vi "Istwerte als Cluster.vi"(8 "error in (no error)":errorcluster caption="Fehler (Eingang, kein Fehler)", 11 "Steuerung PNS Eingang":refnum<class "Steuerung PNS.lvclass">) -> (0 "error out":errorcluster caption="Fehler (Ausgang)", 2 "Cluster":cluster{"UsrVal":u16[], "Alarm":T1, "Regler":T2}, 3 "Steuerung PNS Ausgang":refnum<class "Steuerung PNS.lvclass">)   [LabVIEW 2020, in "Steuerung PNS.lvclass"]
doc: "Gibt die Istwerte von UsrVal, Regler und Alarme als Cluster zurück.\n(zum schreiben in die FGV PNS Istwerte)\nRIW"
uses:
  Steuerung PNS.lvclass
  Alarme.ctl
  Regler.ctl
  Steuerung PNS.lvclass/Steuerung PNS.ctl
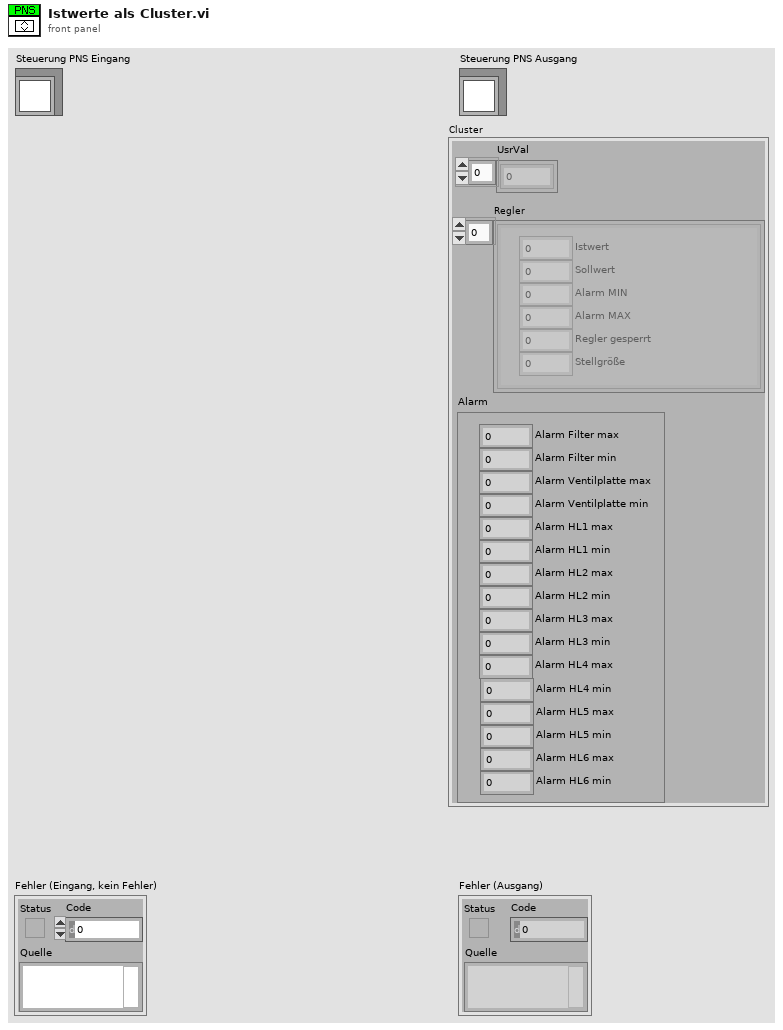
[diagram p1: front panel]
types:
  T1 = typedef "Steuerung PNS.lvclass/Alarme.ctl" = cluster{"Alarm Filter max":u16, "Alarm Filter min":u16, "Alarm Ventilplatte max":u16, "Alarm Ventilplatte min":u16, "Alarm HL1 max":u16, "Alarm HL1 min":u16, "Alarm HL2 max":u16, "Alarm HL2 min":u16, "Alarm HL3 max":u16, "Alarm HL3 min":u16, "Alarm HL4 max":u16, "Alarm HL4 min":u16, "Alarm HL5 max":u16, "Alarm HL5 min":u16, "Alarm HL6 max":u16, "Alarm HL6 min":u16}
  T2 = typedef "Steuerung PNS.lvclass/Regler.ctl" = cluster{"Istwert":i16, "Sollwert":i16, "Alarm MIN":i16, "Alarm MAX":i16, "Regler sperren":i16, "Analog Ausgang":i16}[]
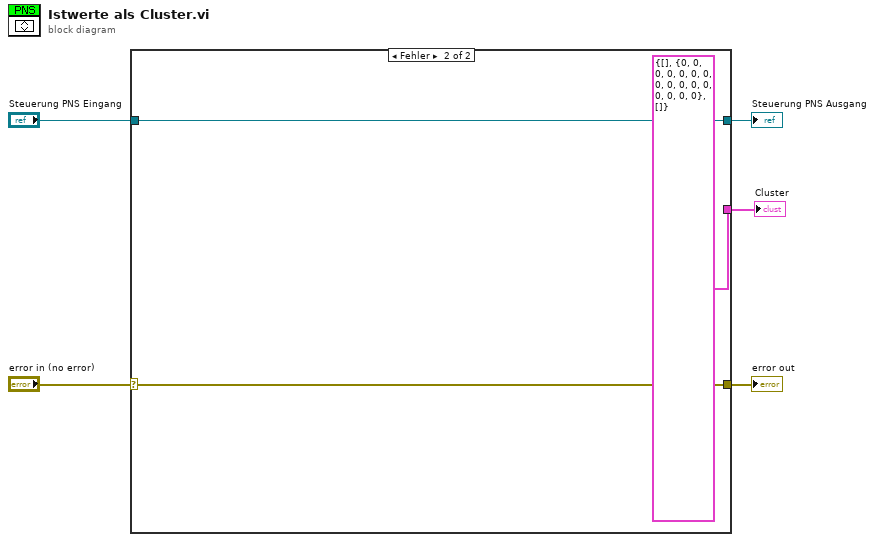
[diagram p0: block diagram]
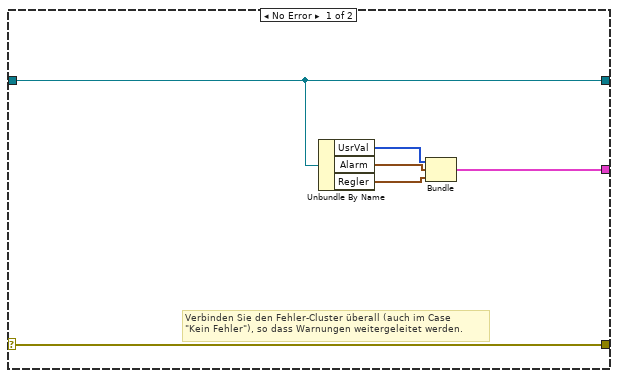
[diagram p2: hidden frame]
diagram:
  n1 = case shown="Fehler" "error in (no error)" {
    selector: "error in (no error)" -> [w11 w14]
    tunnel: [w11 w14] -> w4
    tunnel: [w7 w13] -> w2
    tunnel: "Steuerung PNS Eingang" -> [w7 w13]
    tunnel: [w6 cluster{"UsrVal":u16[], "Alarm":T1, "Regler":T2} {"UsrVal"=[], "Alarm"={"Alarm Filter max"=0, "Alarm Filter min"=0, "Alarm Ventilplatte max"=0, "Alarm Ventilplatte min"=0, "Alarm HL1 max"=0, "Alarm HL1 min"=0, "Alarm HL2 max"=0, "Alarm HL2 min"=0, "Alarm HL3 max"=0, "Alarm HL3 min"=0, "Alarm HL4 max"=0, "Alarm HL4 min"=0, "Alarm HL5 max"=0, "Alarm HL5 min"=0, "Alarm HL6 max"=0, "Alarm HL6 min"=0}, "Regler"=[]}] -> w1
    frame No Error {
      # "Verbinden Sie den Fehler-Cluster überall (auch im Case\n\"Kein Fehler\"), so dass Warnungen weitergeleitet werden."
      n2 = Unbundle By Name(w7) -> ("UsrVal"=w10:u16[], "Alarm"=w9:T1, "Regler"=w8:T2)
      n3 = Bundle("UsrVal"=w10, "Alarm"=w9, "Regler"=w8) -> (w6:cluster{"UsrVal":u16[], "Alarm":T1, "Regler":T2})  [unwired: 1 in]
    }
    frame Error {
    }
  }
  "error out" <- w4
  "Steuerung PNS Ausgang" <- w2
  "Cluster" <- w1
